vi "configure.vi"(8 "error in (no error)":errorcluster, 11 "GenericPlugin in":refnum<class "TrajectoryDL110413StraightLine.lvclass">) -> (0 "error out":errorcluster, 3 "GenericPlugin out":refnum<class "TrajectoryDL110413StraightLine.lvclass">)   [LabVIEW 2010, in "TrajectoryDL110413StraightLine.lvclass"]
doc: "The dynamic dispatch version of this VI loads and displays the configuration file associated with the plug-in object. The user modify and save the configuration data."
uses:
  TrajectoryDL110413StraightLine.lvclass
  common/classes/GenericComponent/GenericComponent/GenericComponent.lvclass
panel:
  in  "z offset XPath":string caption="z offset"
  in  "y offset XPath":string caption="y offset"
  in  "x offset XPath":string caption="x offset"
  out "configuration":string
  in  "cancelButton":bool
  in  "okButton":bool
  # "Configure TrajectoryDL110413StraightLine"
  # "XPaths"
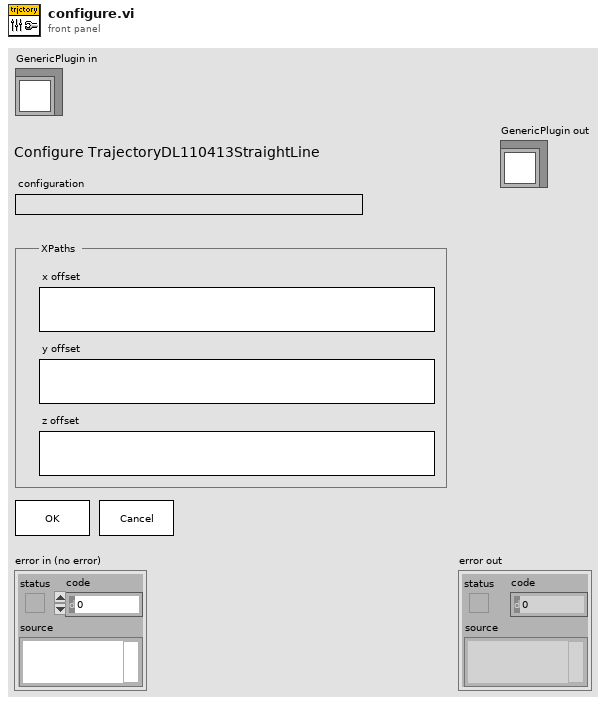
[diagram p1: front panel]
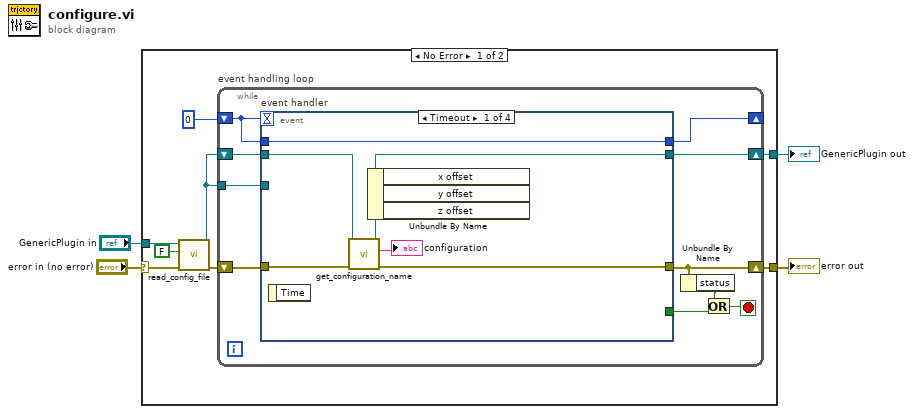
[diagram p0: block diagram]
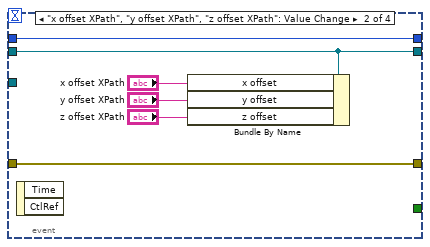
[diagram p2: hidden frame]
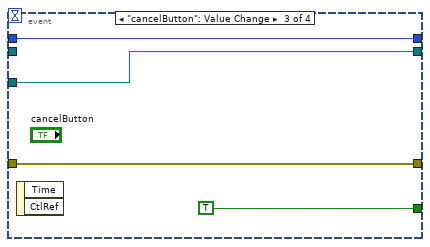
[diagram p3: hidden frame]
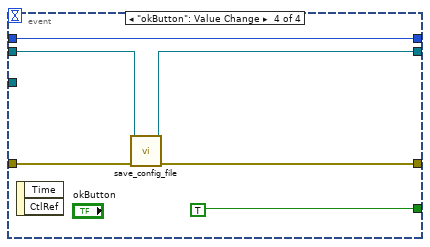
[diagram p4: hidden frame]
diagram:
  n1 = case shown="No Error" "error in (no error)" {
    selector: "error in (no error)" -> [w9 w46]
    tunnel: "GenericPlugin in" -> [w7 w45]
    tunnel: [w11 w46] -> w2
    tunnel: [w12 w45] -> w1
    frame No Error {
      n2 = call-dynamic "read_config_file.vi"("error in (no error)"=w9, "force load?"=FALSE, "GenericPlugin in"=w7) -> ("error out"=w8:errorcluster, "GenericPlugin out"=w6:refnum<class "TrajectoryDL110413StraightLine.lvclass">)  [unwired: 7 in]
      n3 = while "event handling loop" {
        shift-right: [w20] -> w12
        shift-left: w6 -> [w22]
        shift-right: [w19] -> w11
        shift-left: w8 -> [w21]
        shift-right: [w14] -> _
        shift-left: 0 -> [w15]
        tunnel: w6 -> [w13]
        stop <- w16 stop-if-true
        n4 = event "event handler" shown="[0] Timeout" {
          selector: _ -> [_ _ _ _]
          dyn-events: _ -> [_ _ _ _]
          timeout: w15 -> [_ _ _ _]
          tunnel: w22 -> [w27 w32 _ w40]
          tunnel: w21 -> [w25 w34 w38 w42]
          tunnel: [w24 w34 w38 w41] -> w19
          tunnel: [w26 w32 w35 w39] -> w20
          tunnel: [_ _ TRUE TRUE] -> w18
          tunnel: [w28 w33 w36 w43] -> w14
          tunnel: w15 -> [w28 w33 w36 w43]
          tunnel: w13 -> [_ _ w35 _]
          event Timeout {
            n5 = event-data() -> ()  [unwired: 1 in, 1 out]
            n6 = call "get_configuration_name.vi"("error in (no error)"=w25, "GenericPlugin.lvclass in"=w27) -> ("error out"=w24:errorcluster, "configuration name"=→"configuration":string, "GenericPlugin.lvclass out"=w26:refnum<class "TrajectoryDL110413StraightLine.lvclass">)  [unwired: 7 in]
            n7 = Unbundle By Name(w26) -> ()  [unwired: 3 out]
          }
          event "x offset XPath", "y offset XPath", "z offset XPath": Value Change {
            n8 = event-data() -> ()  [unwired: 1 in, 2 out]
            n9 = Bundle By Name(cluster=w32, "x offset"="x offset XPath", "y offset"="y offset XPath", "z offset"="z offset XPath") -> ()  [unwired: 1 out]
          }
          event "cancelButton": Value Change {
            n10 = event-data() -> ()  [unwired: 1 in, 2 out]
          }
          event "okButton": Value Change {
            n11 = event-data() -> ()  [unwired: 1 in, 2 out]
            n12 = call-dynamic "save_config_file.vi"("error in (no error)"=w42, "GenericPlugin in"=w40) -> ("error out"=w41:errorcluster, "GenericPlugin out"=w39:refnum<class "TrajectoryDL110413StraightLine.lvclass">)  [unwired: 8 in]
          }
        }
        n13 = Unbundle By Name(w19) -> ("status"=w17:bool)
        n14 = Or(x=w17, y=w18) -> (x .or. y?=w16:bool)
      }
    }
    frame Error {
    }
  }
  "error out" <- w2
  "GenericPlugin out" <- w1
